vi "AWS-S3-ConstructClient.vi"(5 "Access Key":string, 7 "Secret Key":string, 11 "error in":errorcluster) -> (4 "AWS-S3-API":refnum<class "AWS-S3-API.lvclass">, 15 "error out":errorcluster)   [LabVIEW 2012, in "AWS-S3-API.lvclass"]
uses:
  AWS-S3-API.lvclass
  AWS-S3-Transfer-Progress.ctl
  AWS-S3-Transfer-Header.ctl
  AWS-S3-Transfer-Completed.ctl
  C:/Users/Jack/repo/visualize/Dependencies/aws/AWS-SDK/AWSSDK.dll
  AWS-SDK/AWSSDK.dll
  AWS-S3-API.lvclass/AWS-S3-API.ctl
panel:
  # "Inputs"
  # "Outputs"
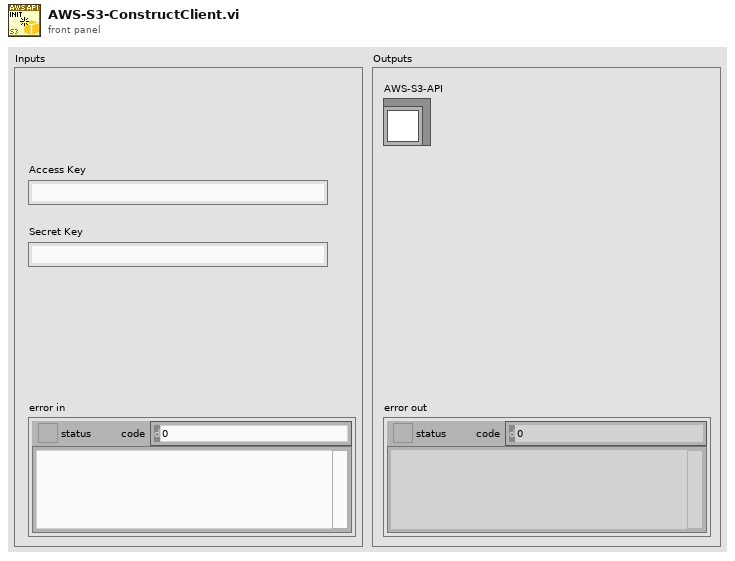
[diagram p1: front panel]
types:
  T1 = typedef "AWS-S3-API.lvclass/AWS-S3-Transfer-Completed.ctl" = cluster{"Transfer Header":T2, "Error?":bool, "Error Message":string}
  T2 = typedef "AWS-S3-API.lvclass/AWS-S3-Transfer-Header.ctl" = cluster{"Bucket Name":string, "Object Name":string, "Local Filepath":path}
  T3 = typedef "AWS-S3-API.lvclass/AWS-S3-Transfer-Progress.ctl" = cluster{"Transfer Header":T2, "Total Bytes":i64, "Transferred Bytes":i64, "Total MB":dbl, "Transferred MB":dbl, "Percent Done (0.0-100.0%)":dbl, "Current Rate (kB/sec)":dbl, "Time Elapsed (sec)":i32, "Est. Time Remaining (sec)":i32}
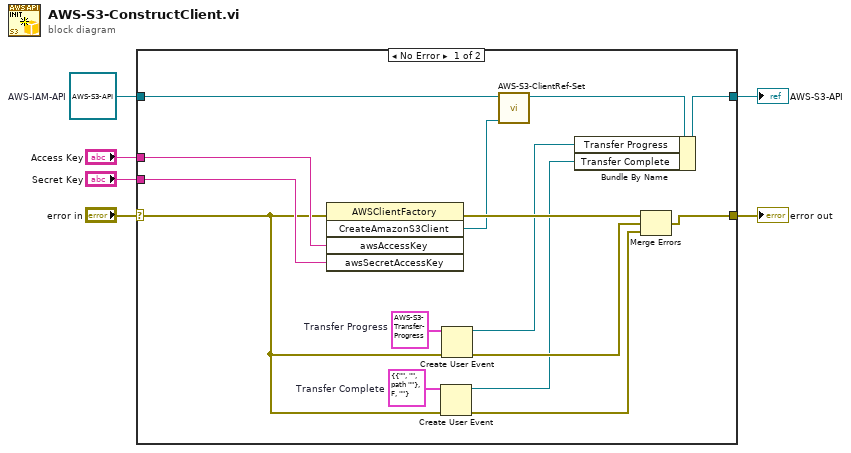
[diagram p0: block diagram]
diagram:
  w5 = refnum<class "AWS-S3-API.lvclass"> refnum  # AWS-IAM-API
  n1 = case shown="No Error" "error in" {
    selector: "error in" -> [w12 w23]
    tunnel: [w16 w23] -> w6
    tunnel: [w21 w22] -> w4
    tunnel: w5 -> [w9 w22]
    tunnel: "Access Key" -> [w20 _]
    tunnel: "Secret Key" -> [w19 _]
    frame No Error {
      w13 = T1 {"Transfer Header"={"Bucket Name"="", "Object Name"="", "Local Filepath"=path ""}, "Error?"=FALSE, "Error Message"=""}  # Transfer Complete
      w18 = T3 {"Transfer Header"={"Bucket Name"="", "Object Name"="", "Local Filepath"=path ""}, "Total Bytes"=0, "Transferred Bytes"=0, "Total MB"=0.0, "Transferred MB"=0.0, "Percent Done (0.0-100.0%)"=0.0, "Current Rate (kB/sec)"=0.0, "Time Elapsed (sec)"=0, "Est. Time Remaining (sec)"=0}  # Transfer Progress
      n2 = invoke class="AWSClientFactory" method="CreateAmazonS3Client"(error in=w12, "awsAccessKey"=w20, "awsSecretAccessKey"=w19) -> (error out=w17:errorcluster, "CreateAmazonS3Client"=w7:refnum<k24>)  [unwired: 2 in, 3 out]
      n3 = Create User Event(user event datatype=w13, error in=w12) -> (user event=w11:refnum<user-event>, error out=w10:errorcluster)
      n4 = Create User Event(user event datatype=w18, error in=w12) -> (user event=w15:refnum<user-event>, error out=w14:errorcluster)
      n5 = call "AWS-S3-ClientRef-Set.vi"("S3 Client ref"=w7, "AWS-S3-API"=w9) -> ("AWS-S3-API out"=w8:refnum<class "AWS-S3-API.lvclass">)  [unwired: 9 in]
      n6 = Bundle By Name(cluster=w8, "Transfer Progress"=w15, "Transfer Complete"=w11) -> (w21:refnum<class "AWS-S3-API.lvclass">)
      n7 = Merge Errors(w17, w14, w10) -> (w16:errorcluster)
    }
    frame Error {
    }
  }
  "error out" <- w6
  "AWS-S3-API" <- w4
